vi "GetValueForKey.vi"() -> ()   [LabVIEW 2018]
panel:
  out "error out":errorcluster
  in  "Key":string="everything"
  in  "Dictionary":cluster{"Key":string, "value":dbl}[](array[cluster])=[{"Key"="test", "value"=123.0}, {"Key"="test2", "value"=456.0}, {"Key"="everything", "value"=42.0}]
  out "value":dbl
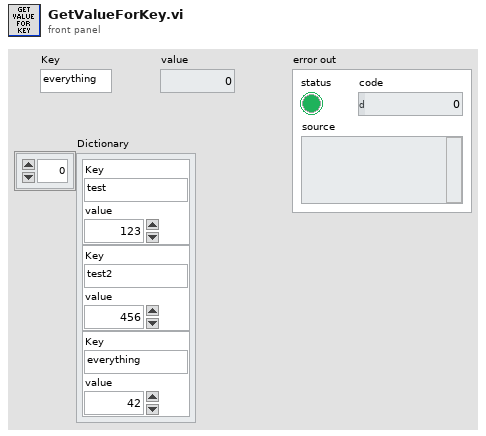
[diagram p1: front panel]
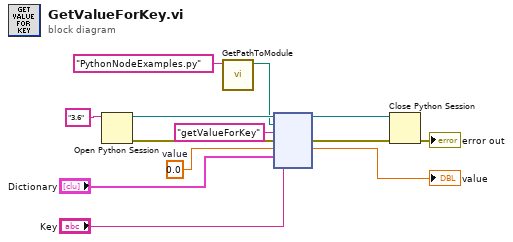
[diagram p0: block diagram]
diagram:
  w7 = 0.0  # value
  n1 = Open Python Session(python version="3.6" ("Python version")) -> (session out=w13:refnum<k35>, error out=w5:errorcluster)  [unwired: 2 in]
  n2 = call "GetPathToModule.vi"("module name"="PythonNodeExamples.py") -> ("path to module"=w1:path)  [unwired: 10 in]
  n3 = node(w13, w1, "getValueForKey" ("function name"), w5, w7, "Dictionary", "Key") -> (w12:refnum<k35>, w4:errorcluster, →"value":dbl)  [unwired: 2 in, 2 out]
  n4 = Close Python Session(session in=w12, error in=w4) -> (11:→"error out":errorcluster)
